vi "Handle Messages.vi"(8 "error in (no error)":errorcluster, 9 "Message Data":variant, 10 "Message":string, 11 "Customer With Phone In":refnum<class "Customer With Phone.lvclass">) -> (0 "error out":errorcluster, 3 "Customer With Phone Out":refnum<class "Customer With Phone.lvclass">)   [LabVIEW 2020, in "Customer With Phone.lvclass"]
uses:
  Customer With Phone.lvclass
  Customer/Customer.lvclass
  Person/Person.lvclass
  C:/Users/anton/Documents/GitHub/Triarc-Examples/Coffee Shop/Processes/People/Customers/Customer/Customer.lvclass
  C:/Users/anton/Documents/GitHub/Triarc-Examples/Coffee Shop/Processes/People/Person/Person.lvclass
  C:/Program Files (x86)/National Instruments/LabVIEW 2020/vi.lib/Asteme/Triarc Framework/View/View.lvclass
  C:/Program Files (x86)/National Instruments/LabVIEW 2020/vi.lib/Asteme/Triarc Framework/Process/Process.lvclass
  C:/Program Files (x86)/National Instruments/LabVIEW 2020/vi.lib/Asteme/Triarc Framework/Base/Base.lvclass
  C:/Program Files (x86)/National Instruments/LabVIEW 2020/vi.lib/Asteme/Triarc Framework/Error Handler Interface/Error Handler Interface.lvclass
  C:/Program Files (x86)/National Instruments/LabVIEW 2020/vi.lib/Asteme/Triarc Framework/Logging/Logging.lvclass
  C:/Users/anton/Documents/GitHub/Triarc-Examples/Coffee Shop/Processes/People/Process Job/Job Handler.lvclass
  C:/Program Files (x86)/National Instruments/LabVIEW 2020/vi.lib/Asteme/Triarc Framework/Asynchronous Action/Async Action.lvclass
  C:/Users/anton/Documents/GitHub/Triarc-Examples/Coffee Shop/Processes/People/Customers/Customer With Phone/Customer With Phone.lvclass
  C:/Program Files (x86)/National Instruments/LabVIEW 2020/vi.lib/Asteme/Triarc Framework/Helper Loop/Helper Loop.lvclass
  <vilib>/Asteme/Triarc Framework/Helper Loop/Helper Loop.lvclass
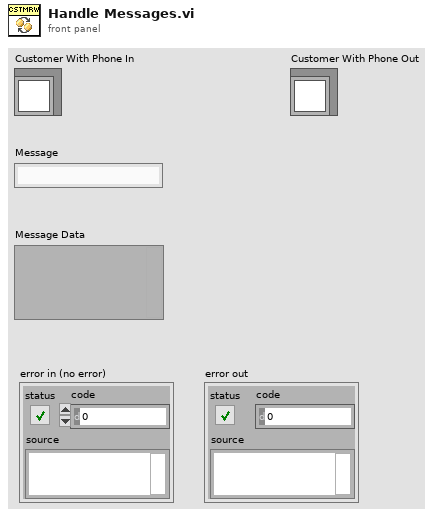
[diagram p1: front panel]
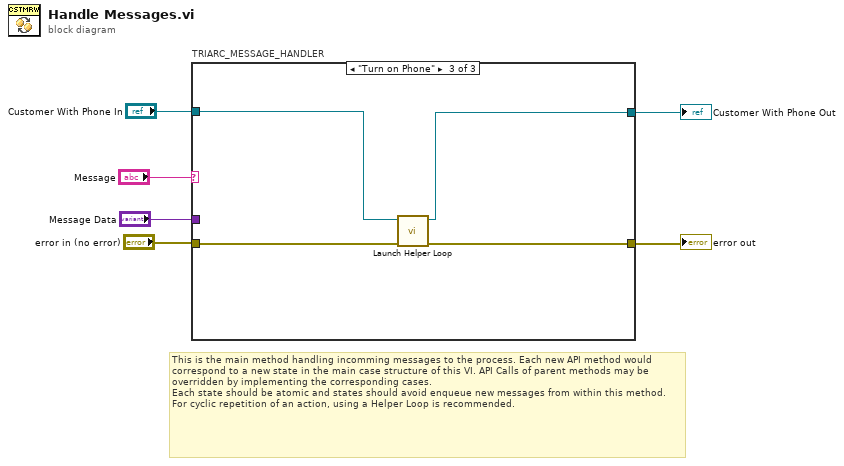
[diagram p0: block diagram]
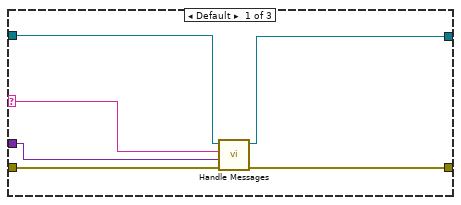
[diagram p2: hidden frame]
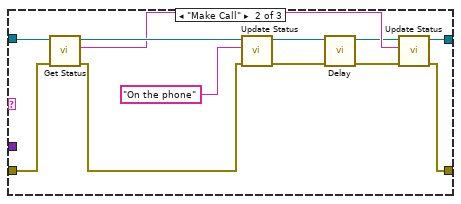
[diagram p3: hidden frame]
diagram:
  # "This is the main method handling incomming messages to the process. Each new API method would correspond to a new state in the main case structure of this VI. API Calls of parent methods may be overridden by implementing the corresponding cases.\nEach state should be atomic and states should avoid enqueue new messages from within this method. For cyclic repetition of an action, using a Helper Loop is recommended."
  n1 = case "TRIARC_MESSAGE_HANDLER" shown="\"Turn on Phone\"" "Message" {
    selector: "Message" -> [w10 _ _]
    tunnel: "error in (no error)" -> [w9 w21 w28]
    tunnel: "Customer With Phone In" -> [w12 w20 w26]
    tunnel: "Message Data" -> [w11 _ _]
    tunnel: [w8 w18 w27] -> w2
    tunnel: [w7 w19 w25] -> w1
    frame Default {
      n2 = call-parent "Handle Messages.vi"("error in (no error)"=w9, "Message Data"=w11, "Message"=w10, "Customer In"=w12) -> ("error out"=w8:errorcluster, "Customer Out"=w7:refnum<class "Customer With Phone.lvclass">)  [unwired: 6 in]
    }
    frame "Make Call" {
      n3 = call "Get Status.vi"("error in (no error)"=w21, "Person In"=w20) -> ("error out"=w22:errorcluster, "Status"=w17:string, "Person Out"=w23:refnum<class "Customer With Phone.lvclass">)  [unwired: 7 in]
      n4 = call "Update Status.vi"("error in (no error)"=w22, "Status"="On the phone", "Person In"=w23) -> ("error out"=w16:errorcluster, "Person Out"=w14:refnum<class "Customer With Phone.lvclass">)  [unwired: 7 in]
      n5 = call "Delay.vi"("error in (no error)"=w16, "Person In"=w14) -> ("error out"=w15:errorcluster, "Person Out"=w13:refnum<class "Customer With Phone.lvclass">)  [unwired: 8 in]
      n6 = call "Update Status.vi"("error in (no error)"=w15, "Status"=w17, "Person In"=w13) -> ("error out"=w18:errorcluster, "Person Out"=w19:refnum<class "Customer With Phone.lvclass">)  [unwired: 7 in]
    }
    frame "Turn on Phone" {
      n7 = call <vilib>:"Launch Helper Loop.vi"("error in (no error)"=w28, "Helper Loop In"=w26) -> ("error out"=w27:errorcluster, "Helper Loop Out"=w25:refnum<class "Customer With Phone.lvclass">)  [unwired: 8 in]
    }
  }
  "error out" <- w2
  "Customer With Phone Out" <- w1
